vi "Memory.Pointer.Write Bytes.vi"   [LabVIEW 2016, in "Memory.Pointer.Void.lvclass"]
uses:
  Memory.Pointer.Void.lvclass
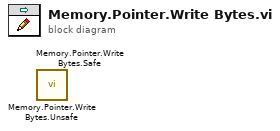
[diagram p0: block diagram]
diagram:
  n1 = call "Memory.Pointer.Write Bytes.Unsafe.vi"() -> ()  [unwired: 8 in, 4 out]
  n2 = call "Memory.Pointer.Write Bytes.Safe.vi"() -> ()  [unwired: 8 in, 4 out]
